vi "11_Demo Voltage Read.vi"(1 "Channel":string="0", 2 "Board ID":i32=1) -> (0 "Measured Voltage":dbl format="%.2f")   [LabVIEW 2016]
doc: "This VI simulates reading voltages from a plug-in data acquisition card. It generates one value at a time from a pre-stored array of values."
panel:
  in  "Readings":i32[](array[numeric])=[163, 163, 163, 163, 163, 163, 165, 169, 172, 173, 172, 172, 171, 171, 174, 176, 177, 178, 178, 179, 178, 177, 176, 175, 175, 174, 173, 172, 172, 172, 172, 172, 171, 171, 170, 170, 170, 172, 173, 174, 175, 177, 178, 178, 178, 177, 176, 175, 176, 178, 179, 180, 179, 178, 178, 176, 176, 176, 174, 174, 174, 173, 173, 175, 176, 178, 178, 177, 176, 175, 175, 174, 174, 173, 173, 172, 172, 171, 171, 170, 170, 170, 170, 170, 170, 170, 169, 166, 167, 169, 170, 169, 168, 168, 168, 168, 167, 167, 167, 167]
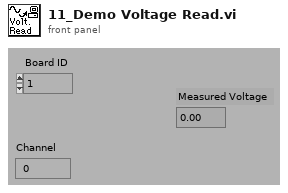
[diagram p1: front panel]
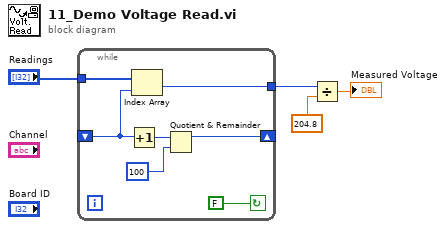
[diagram p0: block diagram]
diagram:
  n1 = while {
    tunnel: "Readings" -> [w6]
    tunnel: [w7] -> w3
    shift-left: _ -> [w11]
    shift-right: [w8] -> _
    stop <- FALSE continue-if-true
    n2 = Increment(x=w11) -> (x+1=w10:i32)
    n3 = Index Array(array=w6, index=w11) -> (element=w7:i32)
    n4 = Quotient & Remainder(x=w10, y=100) -> (x-y*floor(x/y)=w8:i32)  [unwired: 1 out]
  }
  n5 = Divide(x=w3, y=204.8) -> (x/y=→"Measured Voltage":dbl)
